vi "IVIS FRET_Main.vi"() -> ()   [LabVIEW 2021]
doc: "Author: X. Michalet\n(C) 2-23, The Regents of the University of California\n\nSource Code at https://github.com/smXplorer/IVIS-FRET-Analysis"
uses:
  IVIS FRET Parameter.ctl
  IVIS FRET_Time Unit.ctl
  Pictures/Save File Format.ctl
  Image/Image Display Palette Information.ctl
  Image/Image Display Palette Type.ctl
  <vilib>/vision/NI_Vision_Development_Module.lvlib
panel:
  out "Error":errorcluster
  in  "Time Unit:":T1=enum."min"
  in  "Tab Control":T2(tab)
  out "Parameters Graph":cluster{"Time Stamps":dbl[], dbl[]}[](graph)
  out "Frame":i32
  in  "Parameter":T3=enum."f_D E"
  out "Intensity Graph":cluster{"Time Axis":dbl[], "Array":dbl[]}[](graph)
  in  "Display Range":cluster{dbl, dbl}(slide)={0.0, 100.0} scale=0.0..0.2
  in  "Palette":T4(ring)
  in  "Displayed Image":path=path "D:/UCLA Thinkpad Google Drive/Work/Manuscripts/2023/Intensity vs FLI FRET 2023/Figshare Data/Fig 3-5 - Tf-TfR FRET in vivo/IVIS/IVIS data - EXP 192/liver mask label.tif"
  in  "Image Color Scale":dbl(ramp)
  out "Display Image":T5(plugin-control)
  in  "Animated Busy Icon":bool=TRUE
  in  "Background File Name":string="luminescent.TIF"
  in  "g":dbl=0.41 min=0.0
  in  "Liver ROI List":string="DO, AO, FRET"
  in  "UB ROI List":string="DO, AO, FRET"
  in  "Analyze":bool
  in  "Liver Mask":path=path "D:/UCLA Thinkpad Google Drive/Work/Manuscripts/2023/Intensity vs FLI FRET 2023/Figshare Data/Fig 3-5 - Tf-TfR FRET in vivo/IVIS/IVIS data - EXP 192/liver mask label.tif"
  in  "UB Mask":path=path "D:/UCLA Thinkpad Google Drive/Work/Manuscripts/2023/Intensity vs FLI FRET 2023/Figshare Data/Fig 3-5 - Tf-TfR FRET in vivo/IVIS/IVIS data - EXP 192/bladder mask label.tif"
  in  "# Frames":i32=210
  in  "Data Folder Root Name":string="IVIS03_192_"
  in  "Root Folder":path=path "D:/UCLA Thinkpad Google Drive/Work/Manuscripts/2023/Intensity vs FLI FRET 2023/Figshare Data/Fig 3-5 - Tf-TfR FRET in vivo/IVIS/IVIS data - EXP 192"
  # "Quick Start Guide:\n 1. Define the location of the Root Folder (where the data folders are located)\n 2. Define the # Frames\n 3. Define the location of the UB Mask Image\n 4. Define the ROI order as identified in AlliGator, e.g. DO, AO, FRET (mouse)\n 5. Define the location of the liver Mask Image\n 6. Define the ROI order as identified in AlliGator, e.g. DO, AO, FRET (mouse)\n 7. Define gamma\n 8. Specifiy which file to use as background (e.g. luminescent.TIF or readbiasonly.TIF)\n 9. Define which file to display as background image\n10. Run the analysis\n11. Select one of the parameters to display\n12. Move the cursor to select a frame\n13. Adjust the display range (and the palette) to get the parameter map"
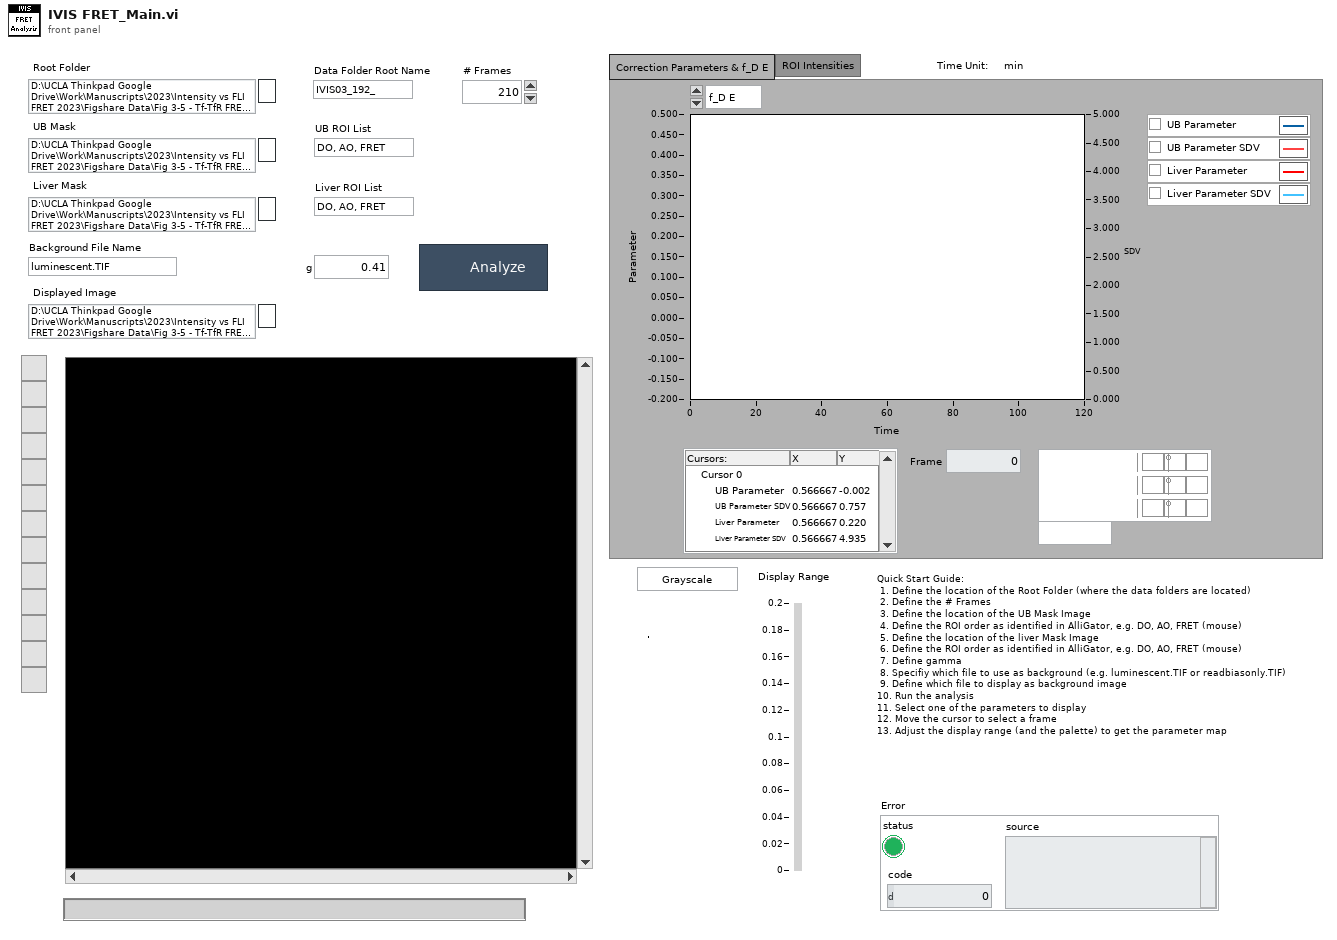
[diagram p1: front panel]
types:
  T1 = typedef "IVIS FRET_Time Unit.ctl" = enum16{"s", "min", "hr"}
  T2 = enum32{"Correction Parameters & f_D E", "ROI Intensities"}
  T3 = typedef "IVIS FRET Parameter.ctl" = enum16{"l_D", "d_D", "l_A", "d_A", "f_D E"}
  T4 = enum16{"Grayscale", "Gradient", "Rainbow", "Temperature"}
  T5 = typedef "IMAQ Image.ctl" = refnum<image>
  T6 = typedef "Save File Format.ctl" = enum16{"PNG", "JPEG", "BMP"}
  T7 = typedef "Image Display Palette Information.ctl" = cluster{"Palette Name [# Colors,int?,inv?]":string, "Palette Type":T8, "Palette Colors":u32[], "Interpolate?":bool}
  T8 = typedef "Image Display Palette Type.ctl" = u32
  T9 = typedef "Image Type" = u32
  T10 = cluster{"l_D":dbl[], "d_D":dbl[], "l_A":dbl[], "d_A":dbl[], "f_D E":dbl[]}[]
  T11 = typedef "Image Point.ctl" = cluster{"X":i32, "Y":i32}
  T12 = cluster{"l_D":dbl[], "d_D":dbl[], "l_A":dbl[], "d_A":dbl[], "f_D E":dbl[]}
  T13 = typedef "IVIS FRET_Frame Image Components.ctl" = cluster{"DD Channel":T5, "AA Channel":T5, "DA Channel":T5}
  T14 = typedef "IVIS FRET_Frame Image Intensities.ctl" = cluster{"DO_DD":dbl, "DO_AA":dbl, "DO_DA":dbl, "AO_DD":dbl, "AO_AA":dbl, "AO_DA":dbl, "DA_DD":dbl, "DA_AA":dbl, "DA_DA":dbl}
  T15 = typedef "IVIS FRET_Series Image Parameter & Coordinates.ctl" = cluster{"[Frame Image Parameters]":cluster{"l_D":dbl[], "d_D":dbl[], "l_A":dbl[], "d_A":dbl[], "f_D E":dbl[]}[], "[DD Pixel Coordinates]":T11[], "[AA Pixel Coordinates]":T11[], "[DA Pixel Coordinates]":T11[]}
  T16 = typedef "IVIS FRET_Frame Image Outputs.ctl" = cluster{"l_D":dbl, "l_D SDV":dbl, "d_D":dbl, "d_D SDV":dbl, "l_A":dbl, "l_A SDV":dbl, "d_A":dbl, "d_A SDV":dbl, "f_D E":dbl, "f_D E SDV":dbl}
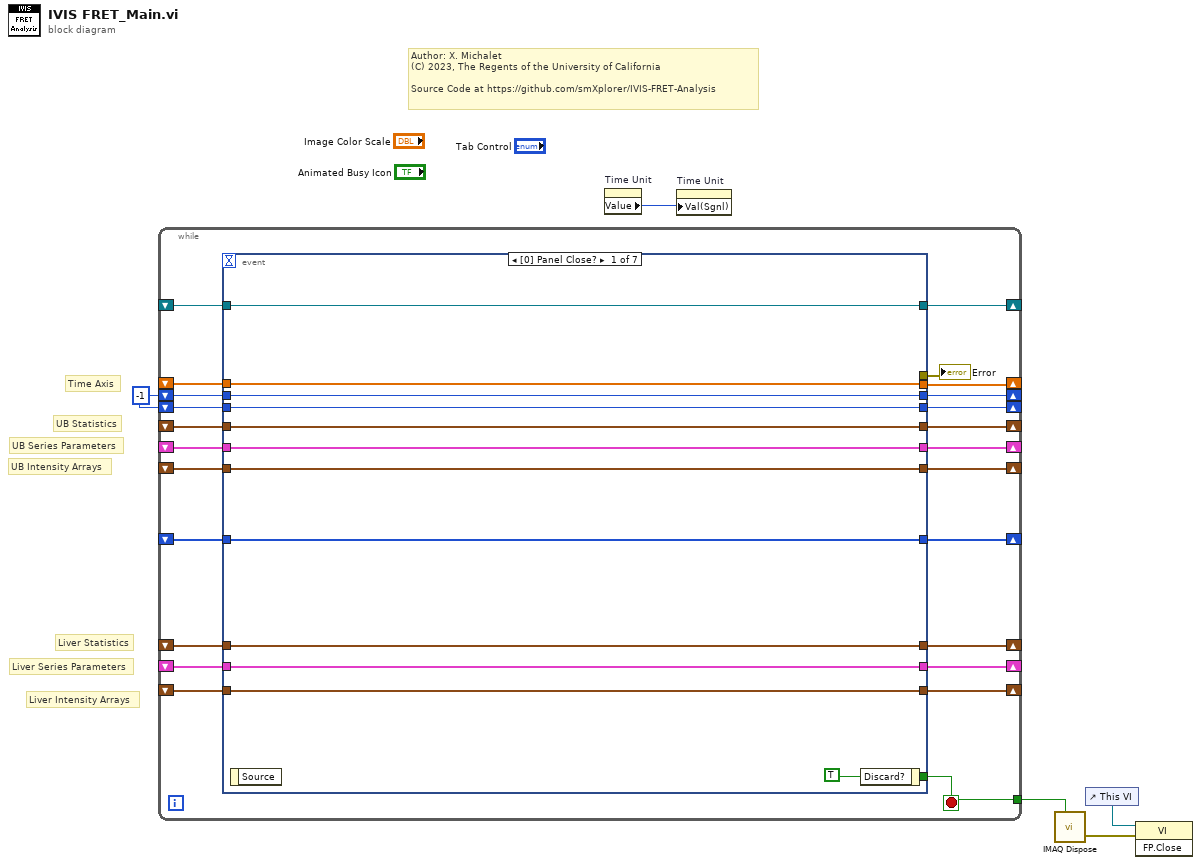
[diagram p0: block diagram]
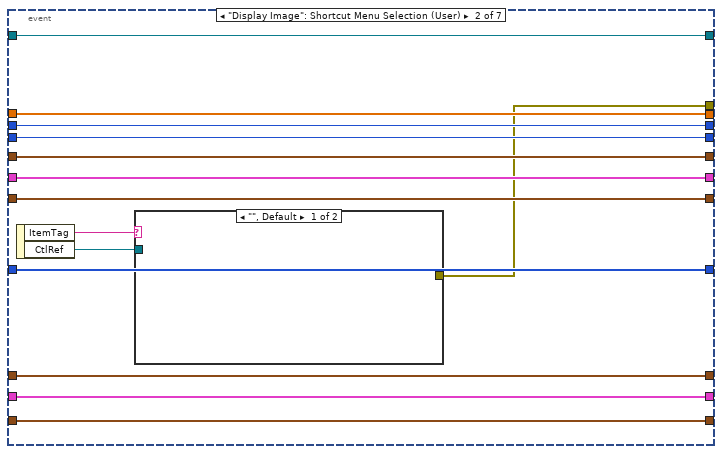
[diagram p2: hidden frame]
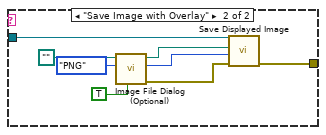
[diagram p3: hidden frame]
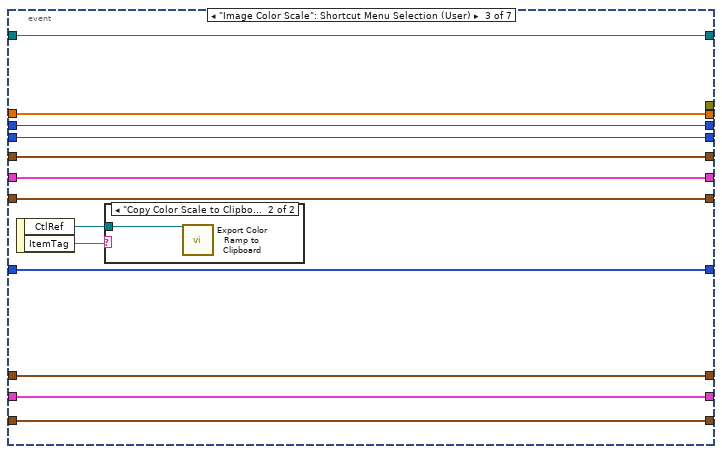
[diagram p4: hidden frame]
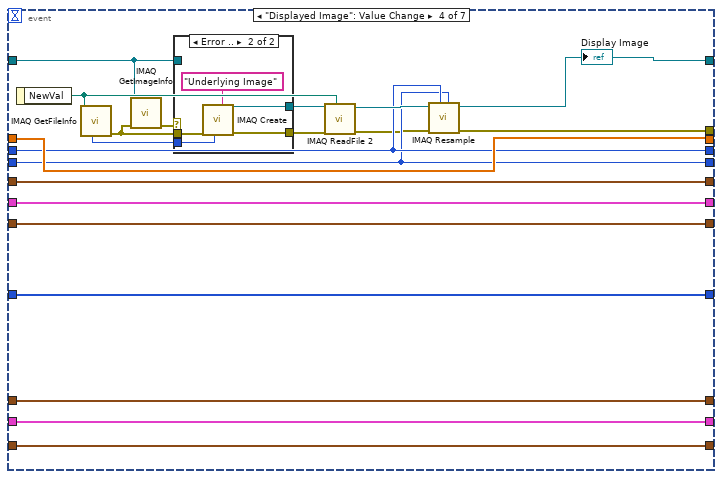
[diagram p6: hidden frame]
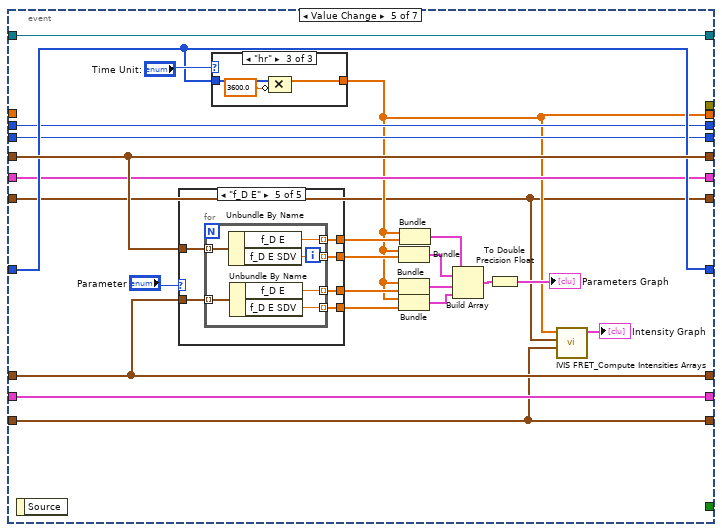
[diagram p8: hidden frame]
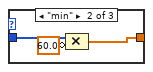
[diagram p10: hidden frame]
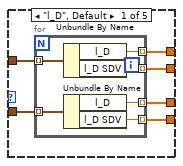
[diagram p11: hidden frame]
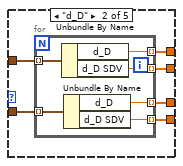
[diagram p12: hidden frame]
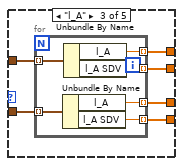
[diagram p13: hidden frame]
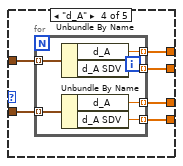
[diagram p14: hidden frame]
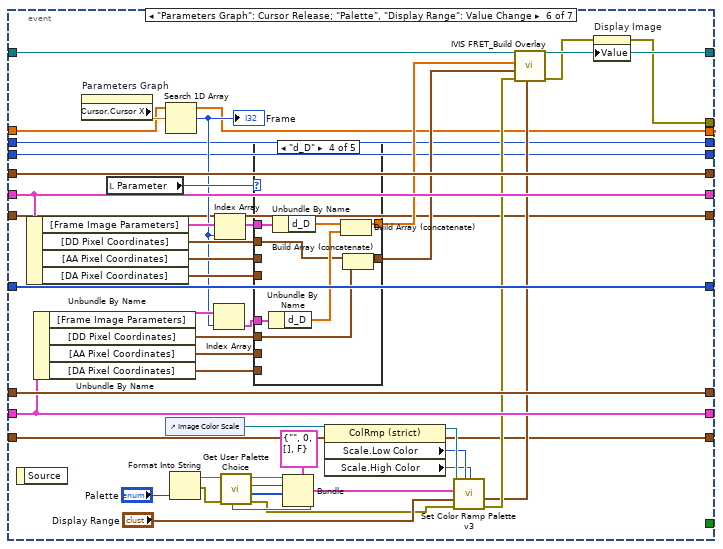
[diagram p15: hidden frame]
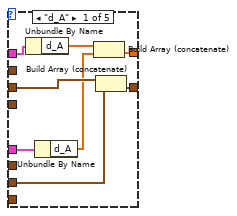
[diagram p16: hidden frame]
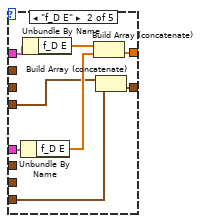
[diagram p17: hidden frame]
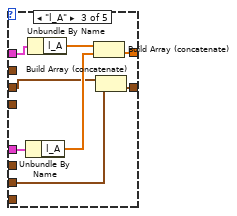
[diagram p18: hidden frame]
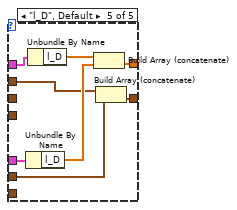
[diagram p19: hidden frame]
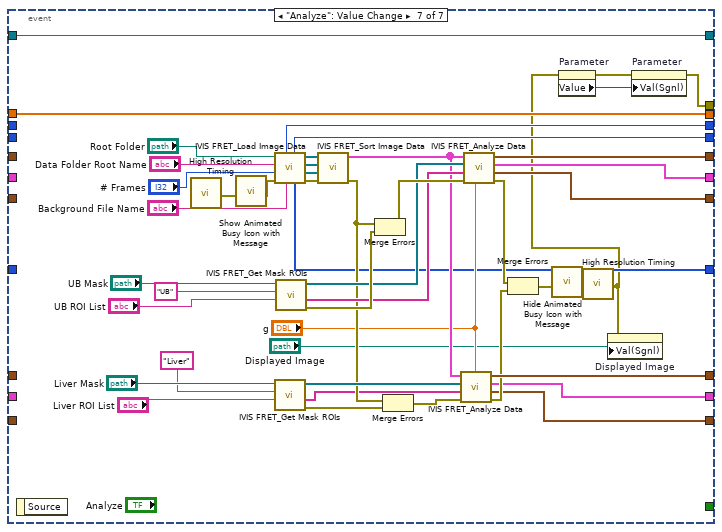
[diagram p20: hidden frame]
diagram:
  w3 = -1 ("X Resolution")
  # "Author: X. Michalet\n(C) 2023, The Regents of the University of California\n\nSource Code at https://github.com/smXplorer/IVIS-FRET-Analysis"
  # "Liver Intensity Arrays"
  # "UB Intensity Arrays"
  # "Time Axis"
  # "Liver Series Parameters"
  # "UB Series Parameters"
  # "Liver Statistics"
  # "UB Statistics"
  n1 = while {
    shift-right: [w29] -> _
    shift-left: _ -> [w26]
    shift-right: [w28] -> _
    shift-left: _ -> [w27]
    tunnel: [w25] -> w5
    shift-right: [w24] -> _
    shift-left: _ -> [w23]
    shift-right: [w21] -> _
    shift-left: _ -> [w22]
    shift-right: [w20] -> _
    shift-left: _ -> [w18]
    shift-right: [w19] -> _
    shift-left: _ -> [w17]
    shift-right: [w16] -> _
    shift-left: _ -> [w15]
    shift-right: [w14] -> _
    shift-left: w3 -> [w12]
    shift-right: [w13] -> _
    shift-left: w3 -> [w11]
    shift-right: [w10] -> _
    shift-left: _ -> [w8]
    shift-right: [w9] -> _
    shift-left: _ -> [w7]
    stop <- w25 stop-if-true
    n2 = event shown="[0] Panel Close?" {
      selector: _ -> [_ _ _ _ _ _ _]
      dyn-events: _ -> [_ _ _ _ _ _ _]
      timeout: _ -> [_ _ _ _ _ _ _]
      tunnel: [w41 _ _ _ _ _ _] -> w25
      tunnel: [w39 w55 w76 w98 w129 w242 w305] -> w29
      tunnel: [w40 w54 w75 w97 w117 w241 w304] -> w28
      tunnel: w27 -> [w40 w54 w75 w97 w117 w241 _]
      tunnel: w26 -> [w39 w55 w76 w98 w129 w242 _]
      tunnel: [w38 w53 w74 w89 w118 w240 w297] -> w24
      tunnel: w23 -> [w38 w53 w74 w89 w118 w240 _]
      tunnel: w22 -> [w37 w52 w73 w90 w116 w239 w294]
      tunnel: [w37 w52 w73 w85 w116 w238 w294] -> w21
      tunnel: [w36 w51 w72 w88 w113 w236 w293] -> w20
      tunnel: [w35 w50 w71 w87 w112 w237 w292] -> w19
      tunnel: w18 -> [w36 w51 w72 w88 w113 w236 _]
      tunnel: w17 -> [w35 w50 w71 w87 w112 w237 _]
      tunnel: [w34 w49 w70 w86 w109 w197 w289] -> w16
      tunnel: w15 -> [w34 w49 w70 w86 _ w197 w289]
      tunnel: [w33 w48 w69 w83 w111 w205 w291] -> w14
      tunnel: [w32 w47 w68 w82 w110 w204 w290] -> w13
      tunnel: w12 -> [w33 w48 w69 w83 w111 w205 _]
      tunnel: w11 -> [w32 w47 w68 w82 w110 w204 _]
      tunnel: [w31 w46 w67 w80 w108 w200 w288] -> w10
      tunnel: [w30 w45 w66 w79 w107 w199 w287] -> w9
      tunnel: w8 -> [w31 w46 w67 w80 w108 w200 _]
      tunnel: w7 -> [w30 w45 w66 w79 w107 w199 _]
      tunnel: [_ w42 _ w78 _ w198 w286] -> w6
      event Panel Close? {
        w41 = TRUE ("Discard?")
        n3 = event-data() -> ()  [unwired: 1 in, 1 out]
        n4 = event-data("Discard?"=w41) -> ()  [unwired: 1 in, 1 out]
      }
      event "Display Image": Shortcut Menu Selection (User) {
        n5 = event-data() -> ("ItemTag"=w44:string, "CtlRef"=w43:refnum<vi>)  [unwired: 1 in]
        n6 = case shown="\"\", Default" w44 {
          tunnel: w43 -> [_ w63]
          tunnel: [_ w56] -> w42
          frame "", Default {
          }
          frame "Save Image with Overlay" {
            n7 = call "Image File Dialog (Optional).vi"("Dialog?"=TRUE, "Image File Format in"=Save_File_Format."PNG", "Default file path in"=path "") -> ("Error Out"=w61:errorcluster, "Image File Format out"=w57:T6, "file path out"=w58:path)  [unwired: 6 in]
            n8 = call "Save Displayed Image.vi"("error in (no error)"=w61, "Saved Image File Format"=w57, "File Path in"=w58, "Display Image Control Refnum"=w63) -> ("Error Out"=w56:errorcluster)  [unwired: 6 in, 1 out]
          }
        }
      }
      event "Image Color Scale": Shortcut Menu Selection (User) {
        n9 = event-data() -> ("CtlRef"=w64:refnum<vi>, "ItemTag"=w65:string)  [unwired: 1 in]
        n10 = case shown="\"Copy Color Scale to Clipboard\"" w65 {
          tunnel: w64 -> [_ w77]
          frame "", Default {
          }
          frame "Copy Color Scale to Clipboard" {
            n11 = call "Export Color Ramp to Clipboard.vi"("ColorRamp in"=w77) -> ()  [unwired: 11 in]
          }
        }
      }
      event "Displayed Image": Value Change {
        n12 = event-data() -> ("NewVal"=w92:path)  [unwired: 1 in]
        n13 = call "IMAQ GetFileInfo"("File Path"=w92) -> ("error out"=w95:errorcluster, "Image Type"=w94:T9)  [unwired: 4 in, 5 out]
        n14 = call "IMAQ GetImageInfo"("error in (no error)"=w95, "Image"=w90) -> ("error out"=w96:errorcluster)  [unwired: 2 in, 7 out]
        n15 = case shown="Error .." w96 {
          tunnel: w95 -> [w100 w105]
          tunnel: w94 -> [_ w104]
          tunnel: [w100 w102] -> w93
          tunnel: [w99 w101] -> w91
          tunnel: w90 -> [w99 _]
          frame No Error {
          }
          frame Error {
            n16 = call "IMAQ Create"("Image Name"="Underlying Image", "Image Type"=w104, "error in (no error)"=w105) -> ("New Image"=w101:T5, "error out"=w102:errorcluster)  [unwired: 2 in]
          }
        }
        n17 = call "IMAQ ReadFile 2"("File Path"=w92, "error in (no error)"=w93, "Image"=w91) -> ("error out"=w81:errorcluster, "Image Out"=w84:T5)  [unwired: 4 in, 3 out]
        n18 = call "IMAQ Resample"("X Resolution"=w82, "Y Resolution"=w83, "error in (no error)"=w81, "Image Src"=w84) -> ("error out"=w78:errorcluster, "Image Dst Out"=w85:T5)  [unwired: 6 in]
        "Display Image" <- w85
      }
      event Value Change {
        n19 = event-data() -> ()  [unwired: 1 in, 1 out]
        n20 = case shown="\"f_D E\"" "Parameter" {
          tunnel: w129 -> [w142 w154 w166 w178 w190]
          tunnel: w117 -> [w141 w153 w165 w177 w189]
          tunnel: [w140 w152 w164 w176 w188] -> w115
          tunnel: [w139 w151 w163 w175 w187] -> w122
          tunnel: [w138 w150 w162 w174 w186] -> w114
          tunnel: [w137 w149 w161 w173 w185] -> w121
          frame "l_D", Default {
            n21 = for {
              tunnel: w142 -> [w148] mode=indexing
              tunnel: w141 -> [w147] mode=indexing
              tunnel: [w146] -> w140 mode=indexing
              tunnel: [w145] -> w139 mode=indexing
              tunnel: [w144] -> w138 mode=indexing
              tunnel: [w143] -> w137 mode=indexing
              n22 = Unbundle By Name(w148) -> ("l_D"=w146:dbl, "l_D SDV"=w145:dbl)
              n23 = Unbundle By Name(w147) -> ("l_D"=w144:dbl, "l_D SDV"=w143:dbl)
            }
          }
          frame "d_D" {
            n24 = for {
              tunnel: w154 -> [w160] mode=indexing
              tunnel: w153 -> [w159] mode=indexing
              tunnel: [w158] -> w152 mode=indexing
              tunnel: [w157] -> w151 mode=indexing
              tunnel: [w156] -> w150 mode=indexing
              tunnel: [w155] -> w149 mode=indexing
              n25 = Unbundle By Name(w160) -> ("d_D"=w158:dbl, "d_D SDV"=w157:dbl)
              n26 = Unbundle By Name(w159) -> ("d_D"=w156:dbl, "d_D SDV"=w155:dbl)
            }
          }
          frame "l_A" {
            n27 = for {
              tunnel: w166 -> [w172] mode=indexing
              tunnel: w165 -> [w171] mode=indexing
              tunnel: [w170] -> w164 mode=indexing
              tunnel: [w169] -> w163 mode=indexing
              tunnel: [w168] -> w162 mode=indexing
              tunnel: [w167] -> w161 mode=indexing
              n28 = Unbundle By Name(w171) -> ("l_A"=w168:dbl, "l_A SDV"=w167:dbl)
              n29 = Unbundle By Name(w172) -> ("l_A"=w170:dbl, "l_A SDV"=w169:dbl)
            }
          }
          frame "d_A" {
            n30 = for {
              tunnel: w178 -> [w184] mode=indexing
              tunnel: w177 -> [w183] mode=indexing
              tunnel: [w182] -> w176 mode=indexing
              tunnel: [w181] -> w175 mode=indexing
              tunnel: [w180] -> w174 mode=indexing
              tunnel: [w179] -> w173 mode=indexing
              n31 = Unbundle By Name(w184) -> ("d_A"=w182:dbl, "d_A SDV"=w181:dbl)
              n32 = Unbundle By Name(w183) -> ("d_A"=w180:dbl, "d_A SDV"=w179:dbl)
            }
          }
          frame "f_D E" {
            n33 = for {
              tunnel: w190 -> [w196] mode=indexing
              tunnel: w189 -> [w195] mode=indexing
              tunnel: [w194] -> w188 mode=indexing
              tunnel: [w193] -> w187 mode=indexing
              tunnel: [w192] -> w186 mode=indexing
              tunnel: [w191] -> w185 mode=indexing
              n34 = Unbundle By Name(w196) -> ("f_D E"=w194:dbl, "f_D E SDV"=w193:dbl)
              n35 = Unbundle By Name(w195) -> ("f_D E"=w192:dbl, "f_D E SDV"=w191:dbl)
            }
          }
        }
        n36 = case shown="\"hr\"" "Time Unit:" {
          tunnel: w118 -> [w130 w133 w136]
          tunnel: [w130 w132 w135] -> w109
          frame "s", Default {
          }
          frame "min" {
            n37 = Compound Arithmetic op=MULTIPLY(w133, invert 60.0 ("value")) -> (w132:dbl[])
          }
          frame "hr" {
            n38 = Compound Arithmetic op=MULTIPLY(w136, invert 3600.0 ("value")) -> (w135:dbl[])
          }
        }
        n39 = Bundle("Time Stamps"=w109, w122) -> (w127:cluster{"Time Stamps":dbl[], dbl[]})  [unwired: 1 in]
        n40 = Bundle("Time Stamps"=w109, w114) -> (w126:cluster{"Time Stamps":dbl[], dbl[]})  [unwired: 1 in]
        n41 = Bundle("Time Stamps"=w109, w121) -> (w125:cluster{"Time Stamps":dbl[], dbl[]})  [unwired: 1 in]
        n42 = Bundle("Time Stamps"=w109, w115) -> (w128:cluster{"Time Stamps":dbl[], dbl[]})  [unwired: 1 in]
        n43 = Build Array(w128, w127, w126, w125) -> (w124:cluster{"Time Stamps":dbl[], dbl[]}[])
        n44 = To Double Precision Float(number=w124) -> (double precision float=→"Parameters Graph":cluster{"Time Stamps":dbl[], dbl[]}[])
        n45 = call "IVIS FRET_Compute Intensities Arrays.vi"("Liver Intensities"=w107, "UB Intensities"=w108, "Time Axis"=w109) -> ("Intensities Arrays"=→"Intensity Graph":cluster{"Time Axis":dbl[], "Array":dbl[]}[])  [unwired: 8 in]
      }
      event "Parameters Graph": Cursor Release; "Palette", "Display Range": Value Change {
        n46 = event-data() -> ()  [unwired: 1 in, 1 out]
        n47 = Unbundle By Name(w236) -> ("[Frame Image Parameters]"=w235:T10, "[DD Pixel Coordinates]"=w223:T11[], "[AA Pixel Coordinates]"=w221:T11[], "[DA Pixel Coordinates]"=w218:T11[])
        n48 = Unbundle By Name(w237) -> ("[Frame Image Parameters]"=w234:T10, "[DD Pixel Coordinates]"=w222:T11[], "[AA Pixel Coordinates]"=w220:T11[], "[DA Pixel Coordinates]"=w219:T11[])
        n49 = property on="Parameters Graph" class="XYGraph (strict)"() -> ("Cursor.Cursor X"=w212:dbl)  [unwired: 2 in, 2 out]
        n50 = local read "Parameter"() -> (w227:T3)
        n51 = Search 1D Array(1D array=w197, element=w212) -> (index of element=w211:i32)  [unwired: 1 in]
        "Frame" <- w211
        n52 = control-ref of="Image Color Scale"() -> (w232:refnum<vi>)
        n53 = Format Into String("Palette") -> (resulting string=w216:string, error out=w214:errorcluster)  [unwired: 3 in]
        n54 = Index Array(array=w234, index=w211) -> (element=w225:T12)
        n55 = Index Array(array=w235, index=w211) -> (element=w226:T12)
        n56 = call "Get User Palette Choice.vi"("Error In"=w214, "Palette"=w216) -> ("Error Out"=w208:errorcluster, "Palette Colors"=w230:u32[], "Palette Type"=w231:T8, "Palette Name (# Colors)"=w228:string, "Interpolate?"=w217:bool)  [unwired: 3 in, 2 out]
        n57 = case shown="\"d_D\"" w227 {
          tunnel: w226 -> [w250 w258 w266 w274 w282]
          tunnel: w225 -> [w249 w257 w265 w273 w281]
          tunnel: [w246 w255 w263 w271 w279] -> w224
          tunnel: w223 -> [_ _ _ w268 w276]
          tunnel: [w244 w253 w261 w269 w277] -> w210
          tunnel: w222 -> [_ _ _ w267 w275]
          tunnel: w221 -> [w247 _ w260 _ _]
          tunnel: w220 -> [w243 _ w259 _ _]
          tunnel: w219 -> [_ w251 _ _ _]
          tunnel: w218 -> [_ w252 _ _ _]
          frame "d_A" {
            n58 = Unbundle By Name(w250) -> ("d_A"=w248:dbl[])
            n59 = Unbundle By Name(w249) -> ("d_A"=w245:dbl[])
            n60 = Build Array (concatenate)(w248, w245) -> (w246:dbl[])
            n61 = Build Array (concatenate)(w247, w243) -> (w244:T11[])
          }
          frame "f_D E" {
            n62 = Unbundle By Name(w257) -> ("f_D E"=w254:dbl[])
            n63 = Unbundle By Name(w258) -> ("f_D E"=w256:dbl[])
            n64 = Build Array (concatenate)(w256, w254) -> (w255:dbl[])
            n65 = Build Array (concatenate)(w252, w251) -> (w253:T11[])
          }
          frame "l_A" {
            n66 = Unbundle By Name(w265) -> ("l_A"=w262:dbl[])
            n67 = Unbundle By Name(w266) -> ("l_A"=w264:dbl[])
            n68 = Build Array (concatenate)(w264, w262) -> (w263:dbl[])
            n69 = Build Array (concatenate)(w260, w259) -> (w261:T11[])
          }
          frame "d_D" {
            n70 = Unbundle By Name(w273) -> ("d_D"=w270:dbl[])
            n71 = Unbundle By Name(w274) -> ("d_D"=w272:dbl[])
            n72 = Build Array (concatenate)(w272, w270) -> (w271:dbl[])
            n73 = Build Array (concatenate)(w268, w267) -> (w269:T11[])
          }
          frame "l_D", Default {
            n74 = Unbundle By Name(w281) -> ("l_D"=w278:dbl[])
            n75 = Unbundle By Name(w282) -> ("l_D"=w280:dbl[])
            n76 = Build Array (concatenate)(w280, w278) -> (w279:dbl[])
            n77 = Build Array (concatenate)(w276, w275) -> (w277:T11[])
          }
        }
        n78 = Bundle(cluster=T7 {"Palette Name [# Colors,int?,inv?]"="", "Palette Type"=0, "Palette Colors"=[], "Interpolate?"=FALSE} ("Image Display Palette Information"), "Palette Name [# Colors,int?,inv?]"=w228, "Palette Type"=w231, "Palette Colors"=w230, "Interpolate?"=w217) -> (w213:T7)
        n79 = property class="ColRmp (strict)"(reference=w232) -> (reference out=w203:refnum<vi>, "Scale.Low Color"=w202:u32, "Scale.High Color"=w201:u32)  [unwired: 1 in, 1 out]
        n80 = call "Set Color Ramp Palette v3.vi"("Image High Color"=w201, "Image Low Color"=w202, "error in (no error)"=w208, "Image Display Range"="Display Range", "Image Display Palette Information"=w213, "ColorRamp in"=w203) -> ("Error Out"=w207:errorcluster, "Scale Marker Values"=w206:cluster{"Numeric":dbl, "Numeric":u32}[])  [unwired: 3 in, 1 out]
        n81 = call "IVIS FRET_Build Overlay.vi"("Color Scale Marker Values"=w206, "Error In"=w207, "[DD Pixel Coordinates]"=w210, "Overlay Values"=w224, "Refnum in"=w239) -> ("Error Out"=w233:errorcluster, "Refnum out"=w238:T5)  [unwired: 5 in]
        n82 = property on="Display Image" class="ImageControl"(error in=w233, "Value"=w238) -> (error out=w198:errorcluster)  [unwired: 1 in, 1 out]
      }
      event "Analyze": Value Change {
        n83 = event-data() -> ()  [unwired: 1 in, 1 out]
        n84 = call "High Resolution Timing.vi"() -> ("Error Out"=w300:errorcluster)  [unwired: 17 in, 2 out]
        n85 = call "Show Animated Busy Icon with Message.vi"("Error In"=w300) -> ("Error Out"=w299:errorcluster)  [unwired: 10 in]
        n86 = call "IVIS FRET_Load Image Data.vi"("Background File Name"="Background File Name", "Error In"=w299, "# Frames"="# Frames", "Data Folder Root Name"="Data Folder Root Name", "Root Folder"="Root Folder") -> ("Error Out"=w321:errorcluster, "[DA Images]"=w322:T5[], "[AA Images]"=w323:T5[], "[DD Images]"=w324:T5[], "Time Stamps"=w297:i64[], "Y Resolution"=w290:i32, "X Resolution"=w291:i32)
        n87 = call "IVIS FRET_Get Mask ROIs.vi"("ROI Type List"="Liver ROI List", "Organ"="Liver", "Mask Image File"="Liver Mask") -> ("error out"=w310:errorcluster, "Ordered ROI Type List"=w307:string[], "Ordered Organ ROI Type Masks"=w311:T5[])  [unwired: 5 in, 1 out]
        n88 = call "IVIS FRET_Get Mask ROIs.vi"("ROI Type List"="UB ROI List", "Organ"="UB", "Mask Image File"="UB Mask") -> ("error out"=w320:errorcluster, "Ordered ROI Type List"=w313:string[], "Ordered Organ ROI Type Masks"=w314:T5[])  [unwired: 5 in, 1 out]
        n89 = call "IVIS FRET_Sort Image Data.vi"("error in (no error)"=w321, "[DA Images]"=w322, "[AA Images]"=w323, "[DD Images]"=w324) -> ("error out"=w308:errorcluster, "Image Array"=w312:T13[])  [unwired: 6 in]
        n90 = Merge Errors(w308, w320) -> (w319:errorcluster)
        n91 = Merge Errors(w308, w310) -> (w309:errorcluster)
        n92 = call "IVIS FRET_Analyze Data.vi"("g"="g", "error in (no error)"=w309, "Ordered ROI Type List"=w307, "Ordered ROI Type Images"=w311, "[Frame Image Data]"=w312) -> ("error out"=w302:errorcluster, "Intensities"=w287:T14[], "Series Parameters & Coordinates"=w292:T15, "[Coeffs & f_D E with SDVs]"=w304:T16[])  [unwired: 3 in]
        n93 = call "IVIS FRET_Analyze Data.vi"("g"="g", "error in (no error)"=w319, "Ordered ROI Type List"=w313, "Ordered ROI Type Images"=w314, "[Frame Image Data]"=w312) -> ("error out"=w303:errorcluster, "Intensities"=w288:T14[], "Series Parameters & Coordinates"=w293:T15, "[Coeffs & f_D E with SDVs]"=w305:T16[])  [unwired: 3 in]
        n94 = Merge Errors(w303, w302) -> (w285:errorcluster)
        n95 = call "Hide Animated Busy Icon with Message.vi"("Error In"=w285) -> ("Error Out"=w298:errorcluster)  [unwired: 10 in]
        n96 = call "High Resolution Timing.vi"("Error In"=w298) -> ("Error Out"=w283:errorcluster)  [unwired: 16 in, 2 out]
        n97 = property on="Parameter" class="Enum (strict)"(error in=w283) -> (error out=w295:errorcluster, "Value"=w296:T3)  [unwired: 1 in, 1 out]
        n98 = property on="Displayed Image" class="Path"(error in=w283, "Val(Sgnl)"="Displayed Image") -> ()  [unwired: 1 in, 2 out]
        n99 = property on="Parameter" class="Enum (strict)"(error in=w295, "Val(Sgnl)"=w296) -> (error out=w286:errorcluster)  [unwired: 1 in, 1 out]
      }
    }
    "Error" <- w6
  }
  n100 = property on="Time Unit" class="Enum (strict)"() -> ("Value"=w4:T1)  [unwired: 2 in, 2 out]
  n101 = property on="Time Unit" class="Enum (strict)"("Val(Sgnl)"=w4) -> ()  [unwired: 2 in, 2 out]
  n102 = call "IMAQ Dispose"("All Images? (No)"=w5) -> ("error out"=w2:errorcluster)  [unwired: 5 in]
  n103 = control-ref of="This VI"() -> (w1:refnum<vi>)
  n104 = invoke class="VI" method="FP.Close"(reference=w1, error in=w2) -> ()  [unwired: 1 in, 3 out]
